vi "test NtripClient-3.vi"() -> ()   [LabVIEW 2019]
uses:
  Ctrl/Ntrip_Account_db.ctl
panel:
  out "hex":string
  out "숫자형":i32
  out "문자열":string
  in  "정지":bool
  out "mount points":string[](array[string])
  out "에러 출력":errorcluster
  in  "Current Ntrip account":T1={"address"="gnss.eseoul.go.kr", "port "=2101, "id"="seoul", "pwd"="seoul", "ref pt"="YONS-RTCM32-M5"}
  out "데이터 출력":string
  in  "read bytes":i32=10000
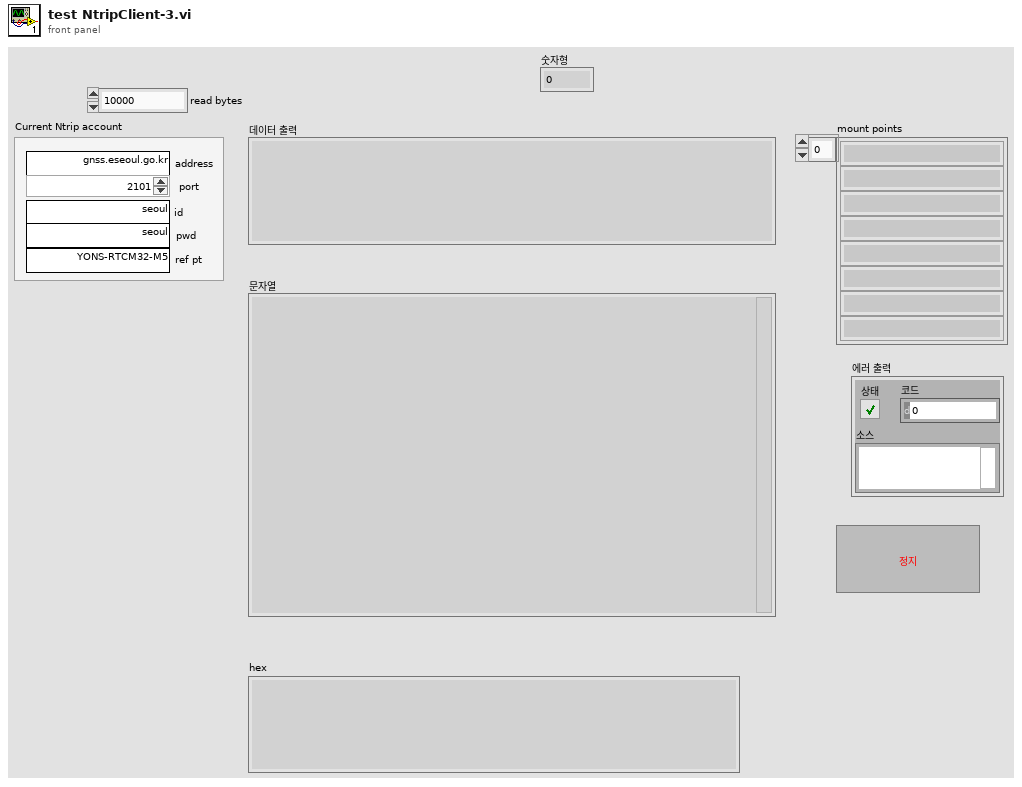
[diagram p1: front panel]
types:
  T1 = typedef "Ntrip_Account_db.ctl" = cluster{"address":string, "port ":u16, "id":string, "pwd":string, "ref pt":string}
  T2 = enum16{"Standard", "Buffered", "CRLF", "Immediate"}
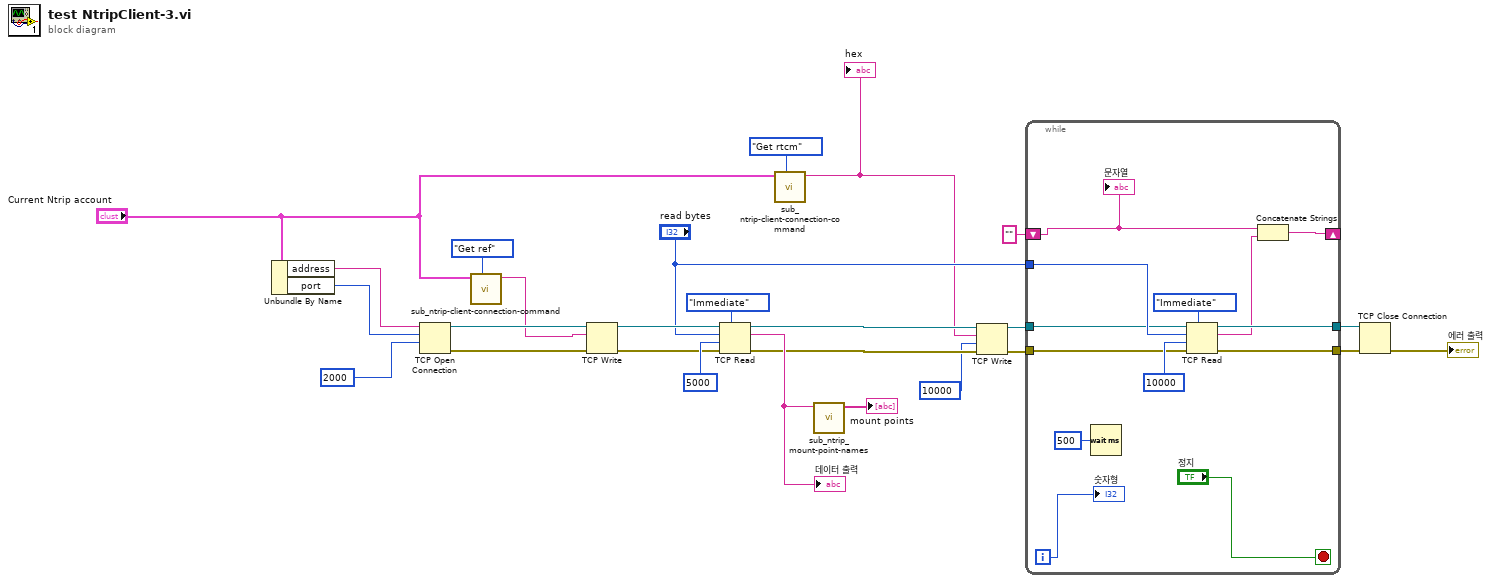
[diagram p0: block diagram]
diagram:
  n1 = Unbundle By Name("Current Ntrip account") -> ("address"=w22:string, "port"=w21:u16)
  n2 = TCP Open Connection(address=w22, remote port or service name=w21, timeout ms (60000)=2000) -> (connection ID=w25:refnum<k5>, error out=w24:errorcluster)  [unwired: 2 in]
  n3 = call "sub_ntrip-client-connection-command.vi"("cmd"=enum16{"Get ref", "Get rtcm"}."Get ref", "Current Ntrip account"="Current Ntrip account") -> ("hex"=w7:string)  [unwired: 9 in]
  n4 = TCP Write(connection ID=w25, data in=w7, error in (no error)=w24) -> (connection ID out=w18:refnum<k5>, error out=w17:errorcluster)  [unwired: 1 in, 1 out]
  n5 = TCP Read(connection ID=w18, bytes to read="read bytes", error in (no error)=w17, 7:T2."Immediate" ("mode (standard)"), 9:5000 ("타임아웃 ms (25000)")) -> (connection ID out=w12:refnum<k5>, data out=w14:string, error out=w11:errorcluster)
  "데이터 출력" <- w14
  n6 = call "sub_ntrip-client-connection-command.vi"("cmd"=enum16{"Get ref", "Get rtcm"}."Get rtcm", "Current Ntrip account"="Current Ntrip account") -> ("hex"=w3:string)  [unwired: 9 in]
  "hex" <- w3
  n7 = call "sub_ntrip_mount-point-names.vi"("ntrip str"=w14) -> ("mount points"=→"mount points":string[])  [unwired: 10 in]
  n8 = TCP Write(connection ID=w12, data in=w3, error in (no error)=w11, 9:10000 ("타임아웃 ms (25000)")) -> (connection ID out=w4:refnum<k5>, error out=w5:errorcluster)  [unwired: 1 out]
  n9 = while {
    tunnel: "read bytes" -> [w37]
    tunnel: w4 -> [w33]
    tunnel: [w38] -> w9
    tunnel: w5 -> [w34]
    tunnel: [w39] -> w10
    shift-right: [w30] -> _
    shift-left: "" -> [w29]
    i -> [w28]
    stop <- "정지" stop-if-true
    n10 = Wait (ms)(milliseconds to wait=u32 500 ("대기 시간 (ms)")) -> ()  [unwired: 1 out]
    n11 = TCP Read(connection ID=w33, bytes to read=w37, error in (no error)=w34, 7:T2."Immediate" ("mode (standard)"), 9:10000 ("타임아웃 ms (25000)")) -> (connection ID out=w38:refnum<k5>, data out=w31:string, error out=w39:errorcluster)
    n12 = Concatenate Strings(w29, w31) -> (w30:string)
    "문자열" <- w29
    "숫자형" <- w28
  }
  n13 = TCP Close Connection(connection ID=w9, error in (no error)=w10) -> (error out=→"에러 출력":errorcluster)  [unwired: 1 in, 1 out]
